vi "Initialize.vi"(7 "Serial Configuration":cluster{"Baud Rate":u32, "Flow Control":u16}={"Baud Rate"=460800, "Flow Control"=0} {"Flow Control" items=["None", "XON/XOFF", "RTS/CTS", "XON/XOFF & RTS/CTS", "DTR/DSR", "XON/XOFF & DTR/DSR"]; "Baud Rate" items=["9600"=9600, "19200"=19200, "38400"=38400, "57600"=57600, "115200"=115200, "230400"=230400, "460800"=460800]}, 8 "error in (no error)":errorcluster, 10 "ID Query (True)":bool=TRUE, 11 "VISA resource name":refnum<visa-resource-name>) -> (0 "error out":errorcluster, 3 "VISA resource name out":refnum<visa-resource-name>)   [LabVIEW 2013, in "California Instruments iX Series.lvlib"]
doc: "Establishes communication with the instrument and optionally performs an instrument identification query and/or an instrument reset. It also places the instrument in a default state needed for other instrument driver operations. Therefore, call this VI before calling other instrument driver VIs for this instrument. Generally, you need to call the Initialize VI only once at the beginning of an application."
uses:
  California Instruments iX Series.lvlib
panel:
  # "(c) 2009 National Instruments.  ALL RIGHTS RESERVED."
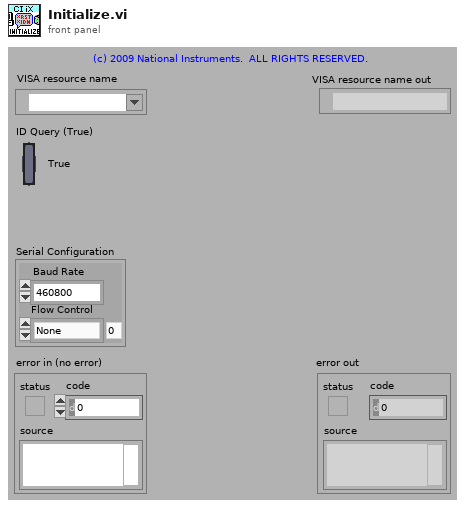
[diagram p1: front panel]
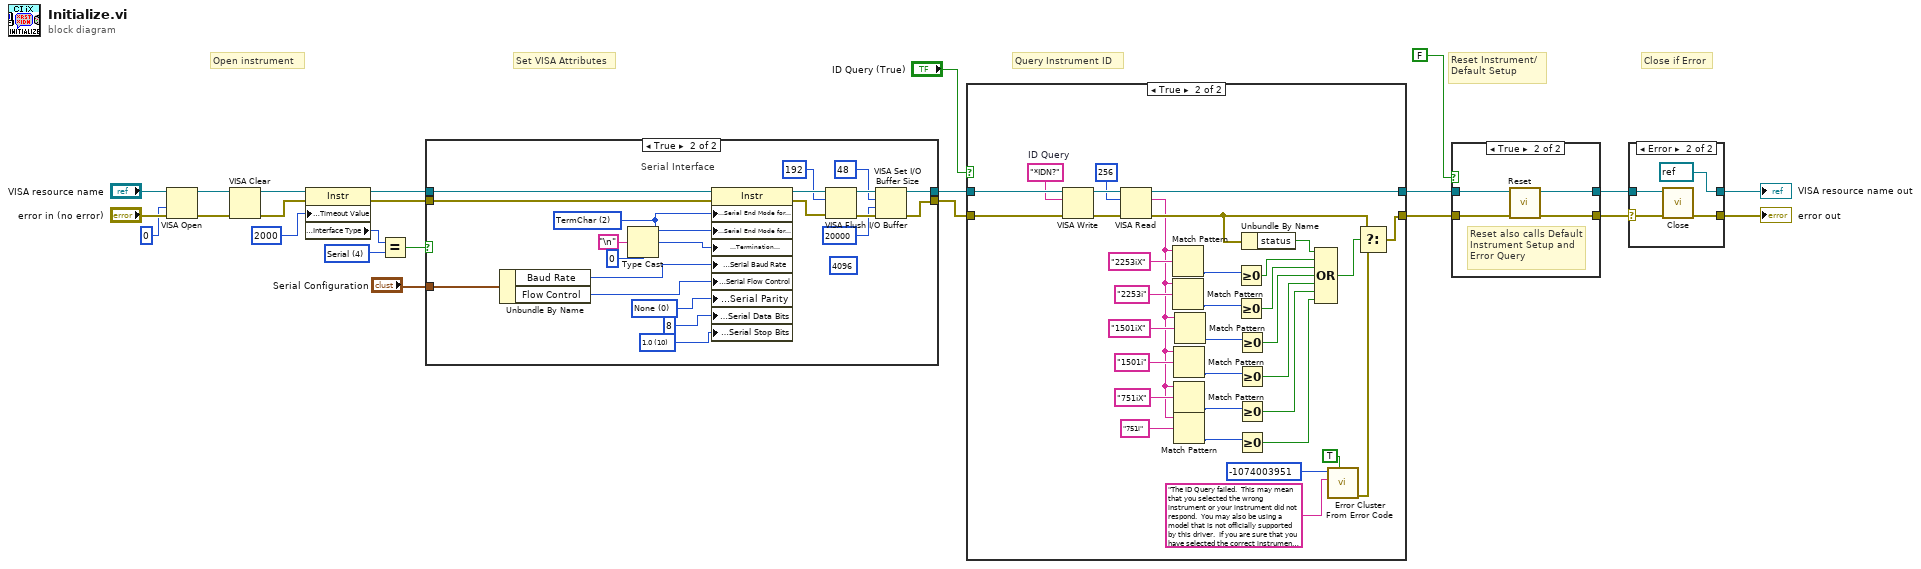
[diagram p0: block diagram]
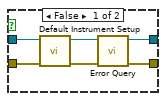
[diagram p4: hidden frame]
diagram:
  w11 = u16 4 items=["GPIB"=1, "VXI"=2, "GPIB-VXI"=3, "Serial"=4, "PXI"=5, "TCPIP"=6, "USB"=7] ("Interface Information:Interface Type")
  # "Set VISA Attributes"
  # "Close if Error"
  # "Query Instrument ID"
  # "Reset Instrument/\nDefault Setup"
  # "Open instrument"
  n1 = VISA Open(access mode=u32 0, error in (no error)="error in (no error)", VISA resource name="VISA resource name") -> (VISA resource name=w9:refnum<visa-resource-name>, error out=w8:errorcluster)  [unwired: 2 in]
  n2 = VISA Clear(VISA resource name=w9, error in (no error)=w8) -> (VISA resource name out=w7:refnum<visa-resource-name>, error out=w6:errorcluster)
  n3 = property class="Instr"(reference=w7, error in=w6, "General Settings:Timeout Value"=u32 2000) -> (reference out=w14:refnum<visa-resource-name>, error out=w13:errorcluster, "Interface Information:Interface Type"=w18:u16)
  n4 = Equal?(x=w18, y=w11) -> (x = y?=w12:bool)
  n5 = case shown="True" w12 {
    tunnel: [w25 w44] -> w16
    tunnel: [w26 w41] -> w15
    tunnel: w14 -> [w25 w46]
    tunnel: w13 -> [w26 w47]
    tunnel: "Serial Configuration" -> [_ w31]
    frame False {
      # "GPIB, TCP/IP, and USB Interface"
    }
    frame True {
      (unwired) u32 4096 ("size (0)")
      w28 = u16 0 items=["None", "Odd", "Even", "Mark", "Space"] ("Serial Settings:Parity")
      w30 = u16 10 items=["1.0"=10, "1.5"=15, "2.0"=20] ("Serial Settings:Stop Bits")
      w35 = u16 2 items=["None", "LastBit", "TermChar"] ("Serial Settings:Serial End Mode for Reads")
      # "Serial Interface"
      n6 = Unbundle By Name(w31) -> ("Baud Rate"=w33:u32, "Flow Control"=w32:u16)
      n7 = Type Cast(type=u8 0, x="\n" ("Line Feed Constant")) -> (*(type *) &x=w34:u8)
      n8 = property class="Instr"(reference=w46, error in=w47, "Serial Settings:Serial End Mode for Reads"=w35, "Serial Settings:Serial End Mode for Writes"=w35, "Message Based Settings:Termination Character"=w34, "Serial Settings:Serial Baud Rate"=w33, "Serial Settings:Serial Flow Control"=w32, "Serial Settings:Serial Parity"=w28, "Serial Settings:Serial Data Bits"=u16 8 ("Serial Settings:Data Bits"), "Serial Settings:Serial Stop Bits"=w30) -> (reference out=w40:refnum<visa-resource-name>, error out=w43:errorcluster)
      n9 = VISA Flush I/O Buffer(VISA resource name=w40, mask (16)=u16 192, error in (no error)=w43) -> (VISA resource name out=w45:refnum<visa-resource-name>, error out=w42:errorcluster)
      n10 = VISA Set I/O Buffer Size(VISA resource name=w45, mask (16)=u16 48, size (4096)=u32 20000 ("size (0)"), error in (no error)=w42) -> (VISA resource name out=w44:refnum<visa-resource-name>, error out=w41:errorcluster)
    }
  }
  n11 = case shown="True" "ID Query (True)" {
    tunnel: [w48 w83] -> w23
    tunnel: [w49 w80] -> w24
    tunnel: w16 -> [w49 w81]
    tunnel: w15 -> [w48 w82]
    frame False {
    }
    frame True {
      w76 = "*IDN?"  # ID Query
      n12 = VISA Write(VISA resource name=w81, write buffer=w76, error in (no error)=w82) -> (VISA resource name out=w79:refnum<visa-resource-name>, error out=w78:errorcluster)  [unwired: 1 out]
      n13 = VISA Read(VISA resource name=w79, byte count=u32 256, error in (no error)=w78) -> (VISA resource name out=w80:refnum<visa-resource-name>, read buffer=w50:string, error out=w71:errorcluster)  [unwired: 1 out]
      n14 = Match Pattern(string=w50, regular expression="2253iX") -> (offset past match=w67:i32)  [unwired: 1 in, 3 out]
      n15 = Match Pattern(string=w50, regular expression="2253i") -> (offset past match=w64:i32)  [unwired: 1 in, 3 out]
      n16 = Match Pattern(string=w50, regular expression="1501i") -> (offset past match=w60:i32)  [unwired: 1 in, 3 out]
      n17 = Match Pattern(string=w50, regular expression="751iX") -> (offset past match=w59:i32)  [unwired: 1 in, 3 out]
      n18 = Match Pattern(string=w50, regular expression="751i") -> (offset past match=w56:i32)  [unwired: 1 in, 3 out]
      n19 = Match Pattern(string=w50, regular expression="1501iX") -> (offset past match=w63:i32)  [unwired: 1 in, 3 out]
      n20 = Greater Or Equal To 0?(x=w67) -> (x >= 0?=w69:bool)
      n21 = Greater Or Equal To 0?(x=w64) -> (x >= 0?=w55:bool)
      n22 = Greater Or Equal To 0?(x=w63) -> (x >= 0?=w54:bool)
      n23 = Greater Or Equal To 0?(x=w60) -> (x >= 0?=w53:bool)
      n24 = Greater Or Equal To 0?(x=w59) -> (x >= 0?=w52:bool)
      n25 = Greater Or Equal To 0?(x=w56) -> (x >= 0?=w51:bool)
      n26 = Unbundle By Name(w71) -> ("status"=w70:bool)
      n27 = Compound Arithmetic op=OR(w70, w69, w55, w54, w53, w52, w51) -> (w68:bool)
      n28 = call <vilib>:"Error Cluster From Error Code.vi"("show call chain? (False)"=TRUE, "error message (\"\")"="The ID Query failed.  This may mean that you selected the wrong instrument or your instrument did not respond.  You may also be using a model that is not officially supported by this driver.  If you are sure that you have selected the correct instrument and it is responding, try disabling the ID Query." ("Source (VI Name)"), "error code (0)"=-1074003951 ("Code")) -> ("error out"=w75:errorcluster)  [unwired: 6 in]
      n29 = Select(t=w71, s=w68, f=w75) -> (s? t:f=w83:errorcluster)
    }
  }
  n30 = case shown="True" FALSE ("Reset (True)") {
    tunnel: w23 -> [w86 w90]
    tunnel: [w88 w93] -> w2
    tunnel: w24 -> [w87 w91]
    tunnel: [w89 w92] -> w3
    frame False {
      n31 = call "Default Instrument Setup.vi"("error in (no error)"=w86, "VISA resource name"=w87) -> ("error out"=w84:errorcluster, "VISA resource name out"=w85:refnum<visa-resource-name>)  [unwired: 8 in]
      n32 = call "Error Query.vi"("error in (no error)"=w84, "VISA resource name"=w85) -> ("error out"=w88:errorcluster, "VISA resource name out"=w89:refnum<visa-resource-name>)  [unwired: 6 in, 2 out]
    }
    frame True {
      # "Reset also calls Default Instrument Setup and Error Query"
      n33 = call "Reset.vi"("error in (no error)"=w90, "VISA resource name"=w91) -> ("error out"=w93:errorcluster, "VISA resource name out"=w92:refnum<visa-resource-name>)  [unwired: 8 in]
    }
  }
  n34 = case shown="Error" w2 {
    selector: w2 -> [w94 w97]
    tunnel: w3 -> [w95 w98]
    tunnel: [w95 refnum<visa-resource-name> refnum ("VISA resource name out")] -> w5
    tunnel: [w94 w99] -> w4
    frame No Error {
    }
    frame Error {
      n35 = call "Close.vi"("error in (no error)"=w97, "VISA resource name"=w98) -> ("error out"=w99:errorcluster)  [unwired: 9 in]
    }
  }
  "VISA resource name out" <- w5
  "error out" <- w4
